vi "HRR-TorqueEnable.vi"(8 "error in":errorcluster, 10 "Enable":bool[](array[boolean]), 11 "FPGA VI Reference In":refnum<k20>) -> (0 "error out":errorcluster, 3 "FPGA VI Reference Out":refnum<k20>)   [LabVIEW 2019]
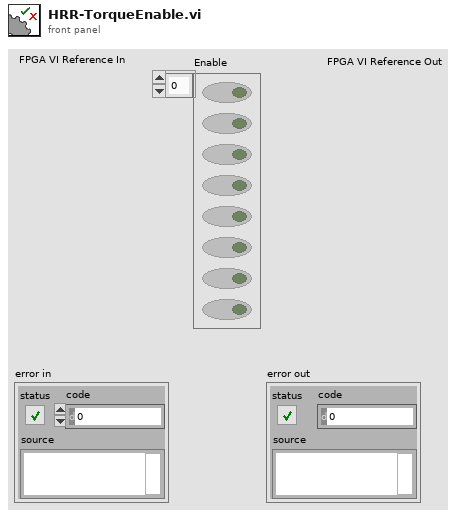
[diagram p1: front panel]
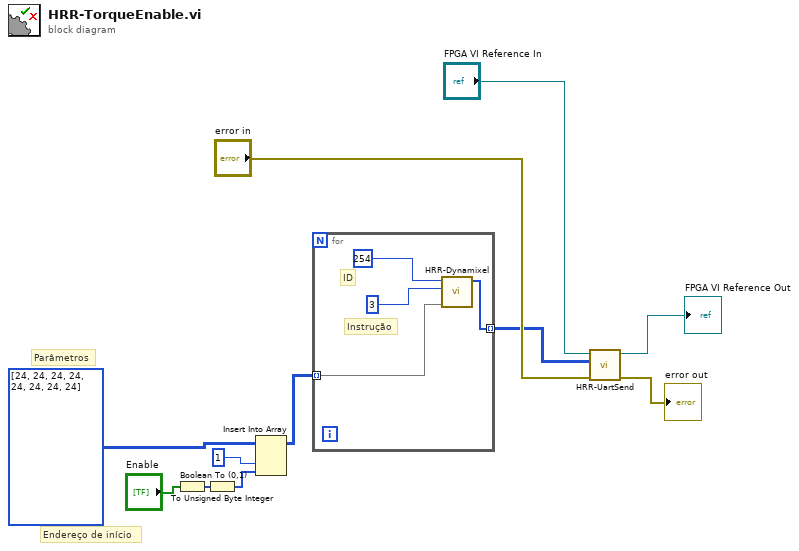
[diagram p0: block diagram]
diagram:
  # "Parâmetros"
  # "Endereço de início"
  n1 = Boolean To (0,1)(Boolean="Enable") -> (0, 1=w2:i16[])
  n2 = To Unsigned Byte Integer(number=w2) -> (unsigned 8bit integer=w1:u8[])
  n3 = Insert Into Array(array=u8[][] [[24], [24], [24], [24], [24], [24], [24], [24]], index (col)=1 ("disabled index (col)"), new element=w1) -> (w7:u8[][])  [unwired: 1 in]
  n4 = for {
    tunnel: w7 -> [w13] mode=indexing
    tunnel: [w12] -> w4 mode=indexing
    # "Instrução"
    # "ID"
    n5 = call "HRR-Dynamixel.vi"("ID"=u8 254, "Instruction"=u8 3, "Array in"=w13) -> ("Array out"=w12:u8[])  [unwired: 7 in]
  }
  n6 = call "HRR-UartSend.vi"("error in (no error)"="error in", "Array"=w4, "Refnum in"="FPGA VI Reference In") -> ("error out"=→"error out":errorcluster, "Refnum out"=→"FPGA VI Reference Out":refnum<k20>)  [unwired: 7 in]
